vi "triggerReadout.vi"() -> (0 "triggerReadout":u16)   [LabVIEW 2014]
uses:
  <vilib>/rvi/eio/common/nirviEmuTemplateMethod_errors.vi
  <vilib>/eio/EIONode/EIONode.xnode
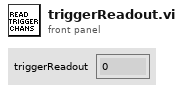
[diagram p1: front panel]
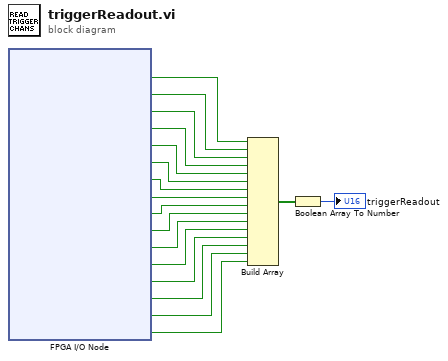
[diagram p0: block diagram]
diagram:
  n1 = xnode "FPGA I/O Node"() -> ("Connector1/DIO24"=w17:bool, "Connector1/DIO25"=w10:bool, "Connector1/DIO26"=w11:bool, "Connector1/DIO27"=w12:bool, "Connector1/DIO28"=w13:bool, "Connector1/DIO29"=w14:bool, "Connector1/DIO30"=w15:bool, "Connector1/DIO31"=w16:bool, "PXI_Trig0"=w9:bool, "PXI_Trig1"=w8:bool, "PXI_Trig2"=w7:bool, "PXI_Trig3"=w6:bool, "PXI_Trig4"=w5:bool, "PXI_Trig5"=w4:bool, "PXI_Trig6"=w3:bool, "PXI_Trig7"=w2:bool)  [unwired: 16 in, 16 out]
  n2 = Build Array(w17, w10, w11, w12, w13, w14, w15, w16, w9, w8, w7, w6, w5, w4, w3, w2) -> (w18:bool[])
  n3 = Boolean Array To Number(Boolean array=w18) -> (number=→"triggerReadout":u16)
